vi "send_main_trigger.vi"(8 "error in (no error)":errorcluster, 10 "trigger":T1) -> (0 "error out":errorcluster)   [LabVIEW 2010]
uses:
  type_definitions/enumerations/main_trigger_enum.ctl
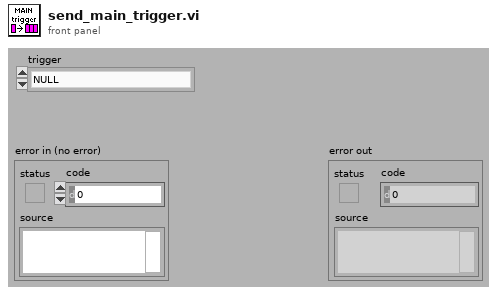
[diagram p1: front panel]
types:
  T1 = typedef "main_trigger_enum.ctl" = enum16{"NULL", "initialise", "terminate", "start", "stop", "change objective", "change experimentController", "change imagingMode", "save notebook", "started saving", "finished saving", "expCtr ready", "expCtr missing", "imgMd ready", "imgMd missing", "scanHd ready", "scanHd missing", "DAQ ready", "DAQ missing", "imgAsm ready", "imgAsm missing", "dataColl ready", "dataColl missing", "display ready", "display missing", "analysr ready", "analysr missing", "instrmnt ready", "instrmnt missing", "stimltr ready", "stimltr missing", "stage ready", "stage missing"}
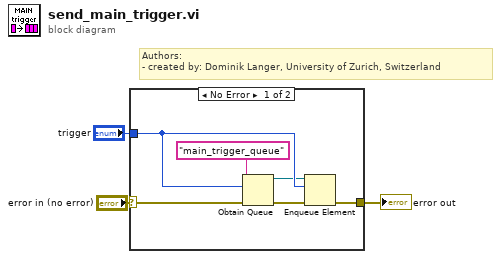
[diagram p0: block diagram]
diagram:
  # "Authors: \n- created by: Dominik Langer, University of Zurich, Switzerland"
  n1 = case shown="No Error" "error in (no error)" {
    selector: "error in (no error)" -> [w9 w10]
    tunnel: "trigger" -> [w7 _]
    tunnel: [w4 w10] -> w1
    frame No Error {
      n2 = Obtain Queue(name (unnamed)="main_trigger_queue", element data type=w7, error in (no error)=w9) -> (queue out=w6:refnum<queue>, error out=w5:errorcluster)  [unwired: 2 in, 1 out]
      n3 = Enqueue Element(queue=w6, element=w7, error in (no error)=w5) -> (error out=w4:errorcluster)  [unwired: 1 in, 2 out]
    }
    frame Error {
    }
  }
  "error out" <- w1
